vi "SetDefaultValue.vi"(6 "error in":errorcluster, 9 "Control Terminal in":refnum<class "ControlTerminal.lvclass">) -> (0 "error out":errorcluster, 3 "Control Terminal out":refnum<class "ControlTerminal.lvclass">, 4 "default":string)   [LabVIEW 2014, in "Raspberry Pi Compatible Compiler for LabVIEW.lvlib" / "ControlTerminal.lvclass"]
uses:
  ControlTerminal.lvclass
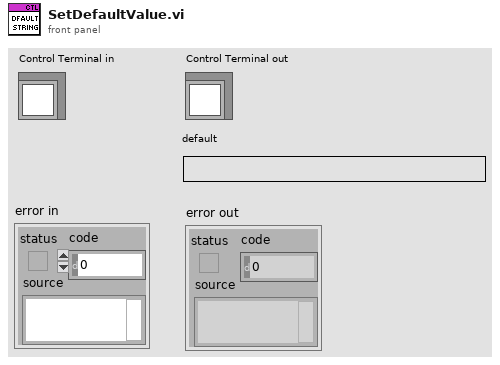
[diagram p1: front panel]
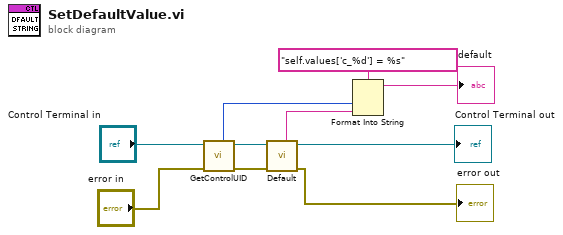
[diagram p0: block diagram]
diagram:
  n1 = call "GetControlUID.vi"("error in"="error in", "Control Terminal in"="Control Terminal in") -> ("error out"=w4:errorcluster, "Control Terminal out"=w5:refnum<class "ControlTerminal.lvclass">, "control UID"=w7:i32)  [unwired: 5 in]
  n2 = call "Default.vi"("error in"=w4, "Control Terminal in"=w5) -> ("error out"=→"error out":errorcluster, "Control Terminal out"=→"Control Terminal out":refnum<class "ControlTerminal.lvclass">, "default"=w6:string)  [unwired: 5 in]
  n3 = Format Into String(format string="self.values['c_%d'] = %s", w7, w6) -> (resulting string=→"default":string)  [unwired: 2 in, 1 out]
